vi "DistanceToTarget.vi"(5 "Image Input":T1=refnum) -> (0 "Y Axis Error":i32=100, 1 "X Axis Error":i32=100, 2 "Object Aquired":bool)   [LabVIEW 2018]
uses:
  <vilib>/vision/Image Controls.llb/IMAQ Image.ctl
panel:
  in  "Pixel Brightness Threshold":i32=250
  in  "Only Scan every nth column":i32=10
  out "Y Location":i32=143
  out "X Location":i32=1050
  out "Brightness of brightest pixel found":i32=100
  in  "Y Max":i32=1180
  in  "X Max":i32=1900
  in  "Y Minimum":i32=20
  in  "X Minimum":i32=20
  # "DistanceToTarget.VI"
  # "Scanning Area:"
  # "Outputs:"
  # "(Distance from Camera FOV Centroid to Laser Dot along X and Y Axes)"
  # "Other Configurations"
  # "This VI currently takes in an image and scans that image for the brightest pixels.  Once those pixels are found - the VI will output the X and Y compnets of a vector that points from the camera's center of view to the tracking target.\n\nIt also has a boolean value, \"Object Aquired\" which is true when there is a pixel brighter than \"Pixel Brightness Threshold\"\n\nThe max possible brightness of any pixel is 255, which correlates to pure white."
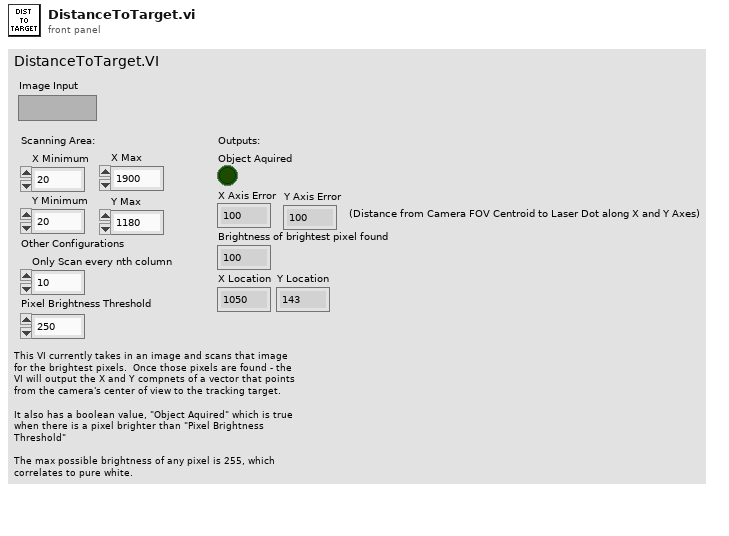
[diagram p1: front panel]
types:
  T1 = typedef "IMAQ Image.ctl" = refnum<image>
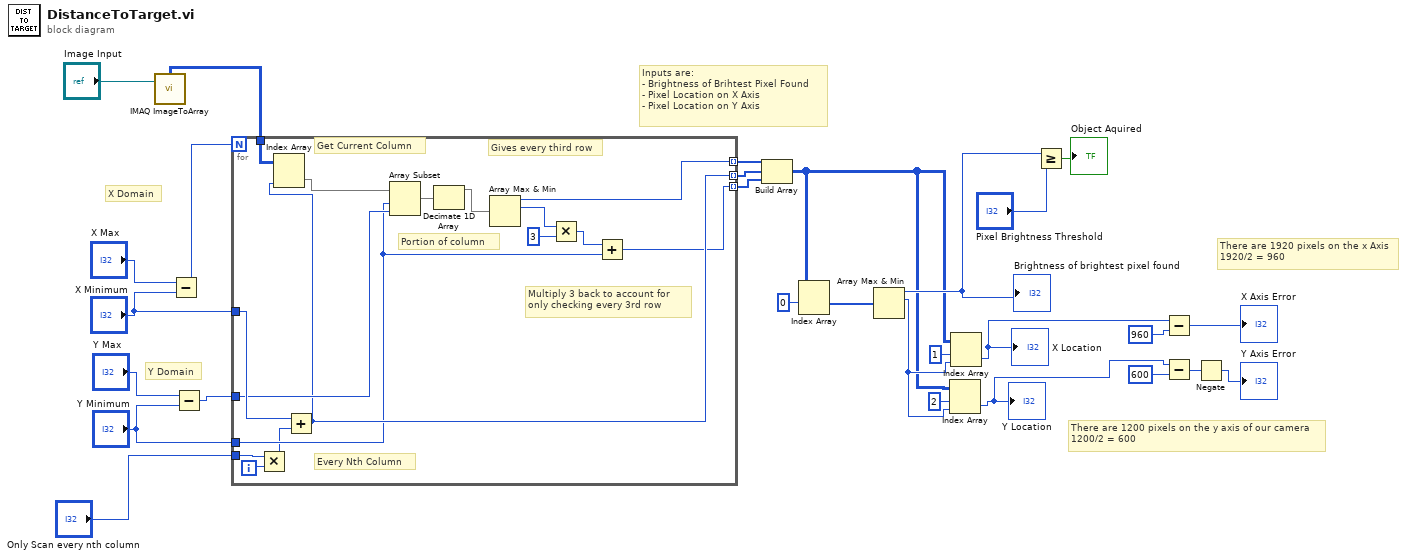
[diagram p0: block diagram]
diagram:
  # "There are 1920 pixels on the x Axis\n1920/2 = 960"
  # "There are 1200 pixels on the y axis of our camera\n1200/2 = 600"
  # "Inputs are:\n- Brightness of Brihtest Pixel Found\n- Pixel Location on X Axis\n- Pixel Location on Y Axis"
  # "Y Domain"
  # "X Domain"
  n1 = call "IMAQ ImageToArray"("Image"="Image Input") -> ("Image Pixels (U8)"=w27:u8[][])  [unwired: 2 in, 5 out]
  n2 = Subtract(x="X Max", y="X Minimum") -> (x-y=w28:i32)
  n3 = Subtract(x="Y Max", y="Y Minimum") -> (x-y=w8:i32)
  n4 = for {
    N: w28 -> [_]
    tunnel: "X Minimum" -> [w44]
    tunnel: w27 -> [w43]
    tunnel: "Y Minimum" -> [w38]
    tunnel: w8 -> [w41]
    tunnel: [w40] -> w26 mode=indexing
    tunnel: [w39] -> w25 mode=indexing
    tunnel: [w37] -> w24 mode=indexing
    tunnel: "Only Scan every nth column" -> [w35]
    i -> [w36]
    # "Multiply 3 back to account for \nonly checking every 3rd row"
    # "Gives every third row"
    # "Every Nth Column"
    # "Portion of column"
    # "Get Current Column"
    n5 = Multiply(x=w35, y=w36) -> (x*y=w34:i32)
    n6 = Add(x=w44, y=w34) -> (x+y=w39:i32)
    n7 = Index Array(array=w43, index (col)=w39) -> (element=w42:u8[])  [unwired: 1 in]
    n8 = Array Subset(array=w42, index=w38, length=w41) -> (w33:u8[])
    n9 = Decimate 1D Array(w33) -> (w32:u8[])  [unwired: 2 out]
    n10 = Array Max & Min(array=w32) -> (max value=w40:u8, max index (indices)=w30:i32)  [unwired: 2 out]
    n11 = Multiply(x=w30, y=3) -> (x*y=w29:i32)
    n12 = Add(x=w29, y=w38) -> (x+y=w37:i32)
  }
  n13 = Build Array(w26, w25, w24) -> (w10:i32[][])
  n14 = Index Array(array=w10, index (row)=0) -> (element=w17:i32[])  [unwired: 1 in]
  n15 = Array Max & Min(array=w17) -> (max value=w12:i32, max index (indices)=w14:i32)  [unwired: 2 out]
  "Brightness of brightest pixel found" <- w12
  n16 = Index Array(array=w10, index (row)=2 ("disabled index (row)"), index (col)=w14) -> (element=w6:i32)
  "Y Location" <- w6
  n17 = Index Array(array=w10, index (row)=1 ("disabled index (row)"), index (col)=w14) -> (element=w4:i32)
  "X Location" <- w4
  n18 = Greater Or Equal?(x=w12, y="Pixel Brightness Threshold") -> (x >= y?=→"Object Aquired":bool)
  n19 = Subtract(x=w4, y=960) -> (x-y=→"X Axis Error":i32)
  n20 = Subtract(x=w6, y=600) -> (x-y=w3:i32)
  n21 = Negate(x=w3) -> (-x=→"Y Axis Error":i32)
